vi "Close.vi"(8 "error in (no error)":errorcluster, 11 "Resource in":refnum<class "Resource.lvclass">) -> (0 "error out":errorcluster, 3 "Resource out":refnum<class "Resource.lvclass">)   [LabVIEW 2020, in "PicoG-Core.lvlib" / "Resource.lvclass"]
uses:
  Resource.lvclass
  Resource.lvclass/Resource.ctl
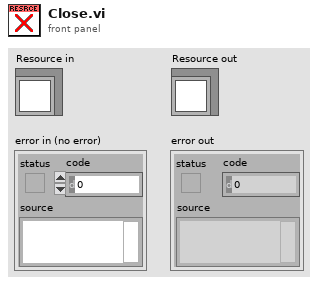
[diagram p1: front panel]
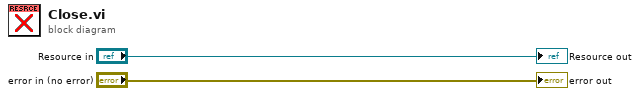
[diagram p0: block diagram]
diagram:
  "error out" <- "error in (no error)"
  "Resource out" <- "Resource in"
